vi "Update State Data.vi"(8 "error in (no error)":errorcluster, 9 "Variant":variant, 10 "Argument":string, 11 "State Data":T1) -> (0 "error out":errorcluster, 3 "State Data out":T1)   [LabVIEW 2020, in "Code Cleanup.lvlib"]
uses:
  Code Cleanup.lvlib
  CTLs/Main State Data.ctl
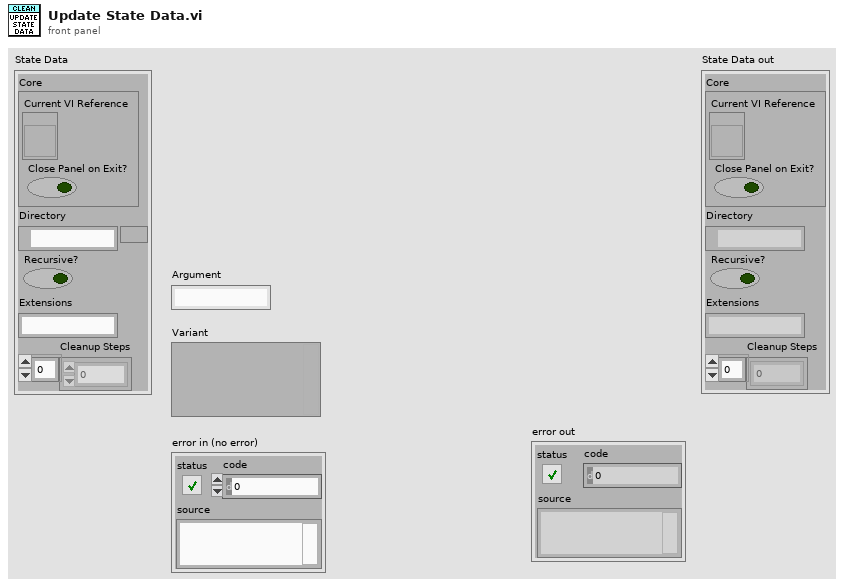
[diagram p1: front panel]
types:
  T1 = typedef "Code Cleanup.lvlib/Main State Data.ctl" = cluster{"Core":cluster{"Current VI Reference":refnum<vi>, "Close Panel on Exit?":bool}, "Directory":path, "Recursive?":bool, "Extensions":string, "Cleanup Steps":i32[]}
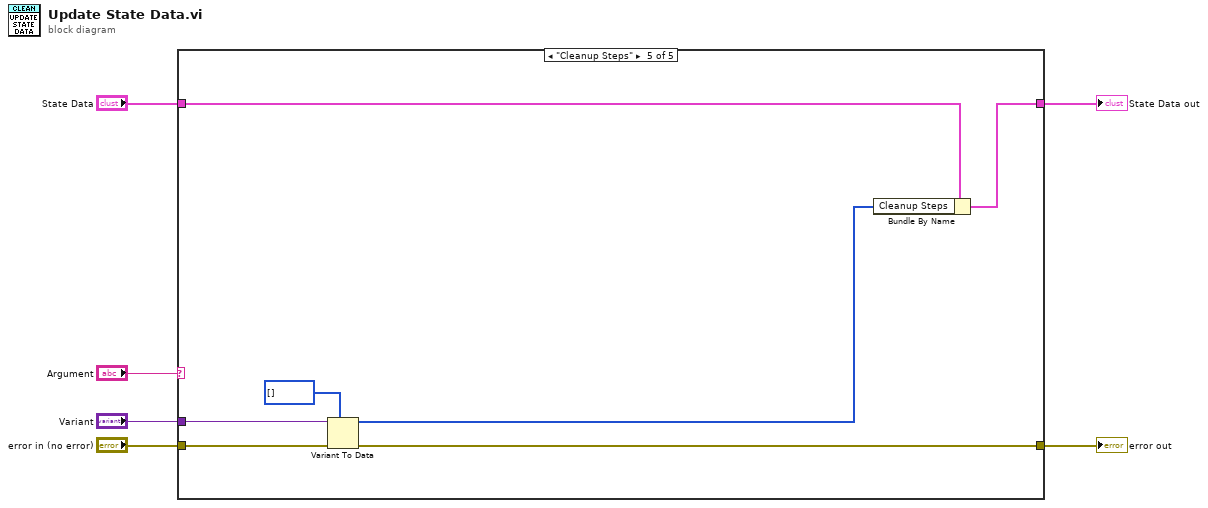
[diagram p0: block diagram]
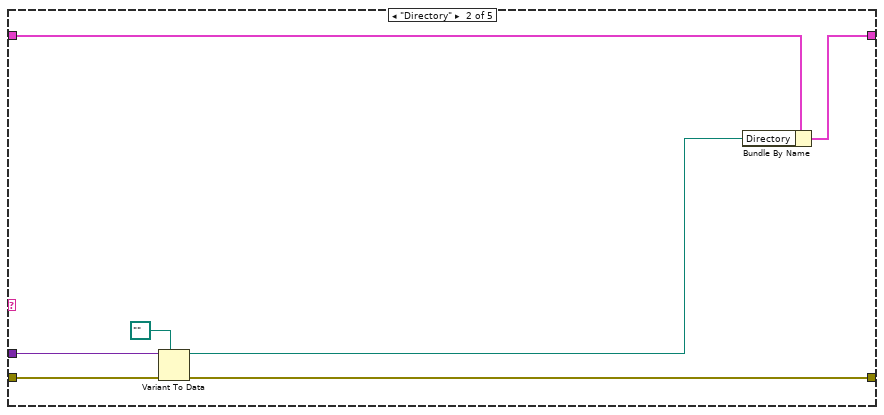
[diagram p3: hidden frame]
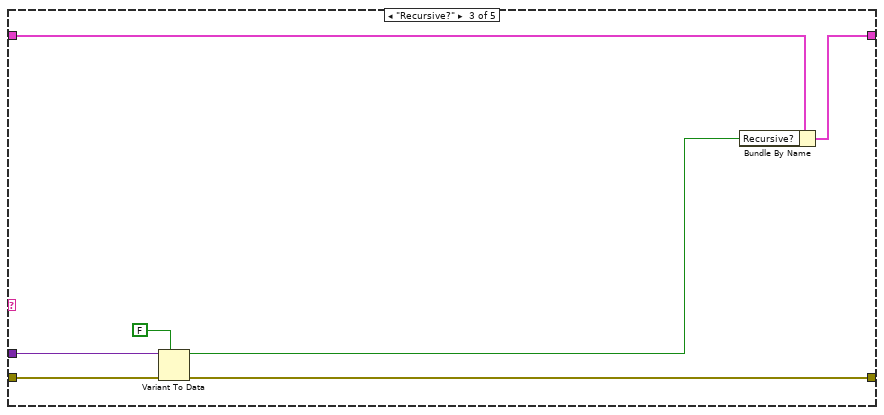
[diagram p4: hidden frame]
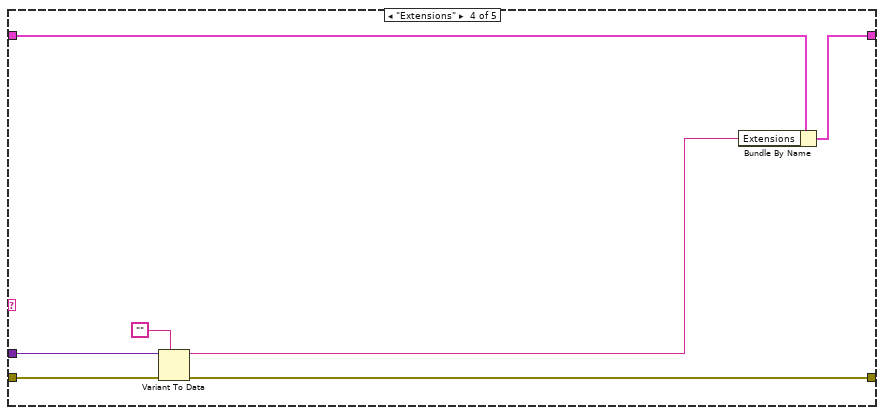
[diagram p5: hidden frame]
diagram:
  n1 = case shown="\"Cleanup Steps\"" "Argument" {
    tunnel: "error in (no error)" -> [w7 w13 w20 w27 w34]
    tunnel: "State Data" -> [w8 w15 w22 w29 w36]
    tunnel: [w8 w14 w21 w28 w35] -> w3
    tunnel: [w7 w10 w17 w24 w32] -> w2
    tunnel: "Variant" -> [_ w12 w19 w26 w33]
    frame Default {
    }
    frame "Directory" {
      n2 = Variant To Data(error in=w13, type=path "", Variant=w12) -> (data=w9:path, error out=w10:errorcluster)
      n3 = Bundle By Name(cluster=w15, "Directory"=w9) -> (w14:T1)
    }
    frame "Recursive?" {
      n4 = Variant To Data(error in=w20, type=FALSE, Variant=w19) -> (data=w16:bool, error out=w17:errorcluster)
      n5 = Bundle By Name(cluster=w22, "Recursive?"=w16) -> (w21:T1)
    }
    frame "Extensions" {
      n6 = Variant To Data(error in=w27, type="", Variant=w26) -> (data=w23:string, error out=w24:errorcluster)
      n7 = Bundle By Name(cluster=w29, "Extensions"=w23) -> (w28:T1)
    }
    frame "Cleanup Steps" {
      n8 = Variant To Data(error in=w34, type=i32[] [], Variant=w33) -> (data=w31:i32[], error out=w32:errorcluster)
      n9 = Bundle By Name(cluster=w36, "Cleanup Steps"=w31) -> (w35:T1)
    }
  }
  "error out" <- w2
  "State Data out" <- w3
